vi "Helmholtz2D_FEM_Assemble.vi"(11 "Helmholtz2D FEM Data In":T1) -> (3 "Helmholtz2D FEM Data Out":T1)   [LabVIEW 2020, in "NI_PDE.lvlib"]
uses:
  <vilib>/gmath/NI_PDE.lvlib
  <vilib>/gmath/pde.llb/Helmholtz2D_FEM/Helmholtz2D_FEM_Data.ctl
  <vilib>/gmath/pde.llb/Common/PDE_Sparse Mtrx.ctl
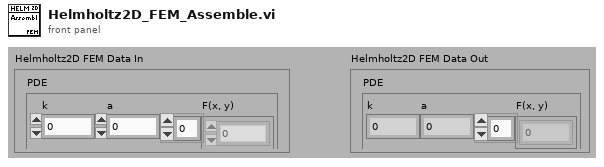
[diagram p1: front panel]
types:
  T1 = typedef "NI_PDE.lvlib/Helmholtz2D_FEM_Data.ctl" = cluster{"PDE":cluster{"k":dbl, "a":dbl, "F(x, y)":dbl[]}, "# of unknown":i32, "# of known":i32, "U(x, y)":dbl[], "X Used":dbl[], "Y Used":dbl[], "Triangulation":i32[][], "Coef Mtrx":T2}
  T2 = typedef "NI_PDE.lvlib/PDE_Sparse Mtrx.ctl" = cluster{"Row":cluster{"col":i32, "value":dbl}[]}[]
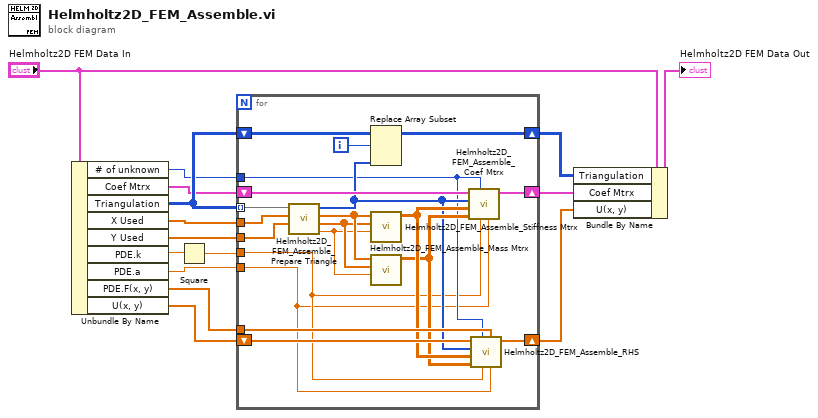
[diagram p0: block diagram]
diagram:
  n1 = Unbundle By Name("Helmholtz2D FEM Data In") -> ("# of unknown"=w11:i32, "Coef Mtrx"=w12:T2, "Triangulation"=w14:i32[][], "X Used"=w15:dbl[], "Y Used"=w13:dbl[], "PDE.k"=w8:dbl, "PDE.a"=w1:dbl, "PDE.F(x, y)"=w10:dbl[], "U(x, y)"=w9:dbl[])
  n2 = Square(x=w8) -> (x^2=w7:dbl)
  n3 = for {
    tunnel: w14 -> [w35] mode=indexing
    tunnel: w15 -> [w34]
    shift-right: [w31] -> w4
    shift-left: w14 -> [w32]
    tunnel: w13 -> [w33]
    shift-right: [w25] -> w3
    shift-left: w12 -> [w26]
    tunnel: w11 -> [w19]
    shift-right: [w16] -> w2
    shift-left: w9 -> [w24]
    tunnel: w10 -> [w23]
    tunnel: w7 -> [w18]
    tunnel: w1 -> [w17]
    i -> [w30]
    n4 = call <vilib>:"Helmholtz2D_FEM_Assemble_Prepare Triangle.vi"("Y"=w33, "X"=w34, "Triangle In"=w35) -> ("area"=w27:dbl, "Tri Y"=w28:dbl[], "Tri X"=w29:dbl[], "Triangle Out"=w20:i32[])  [unwired: 5 out]
    n5 = Replace Array Subset(array=w32, new element=w20, index (row)=w30) -> (w31:i32[][])  [unwired: 1 in]
    n6 = call <vilib>:"Helmholtz2D_FEM_Assemble_Stiffness Mtrx.vi"("area"=w27, "Tri Y"=w28, "Tri X"=w29) -> ("Stiffness Mtrx"=w22:dbl[][])  [unwired: 8 out]
    n7 = call <vilib>:"Helmholtz2D_FEM_Assemble_Mass Mtrx.vi"("area"=w27, "Tri Y"=w28, "Tri X"=w29) -> ("Mass Mtrx"=w21:dbl[][])  [unwired: 8 out]
    n8 = call <vilib>:"Helmholtz2D_FEM_Assemble_Coef Mtrx.vi"("a"=w17, "k"=w18, "# of unknown"=w19, "Mass Mtrx"=w21, "Stiffness Mtrx"=w22, "Triangle"=w20, "Coef Mtrx In"=w26) -> ("Coef Mtrx Out"=w25:T2)  [unwired: 4 out]
    n9 = call <vilib>:"Helmholtz2D_FEM_Assemble_RHS.vi"("a"=w17, "F(x, y)"=w23, "k"=w18, "# of unknown"=w19, "Mass Mtrx"=w21, "Stiffness Mtrx"=w22, "Triangle"=w20, "RHS In"=w24) -> ("RHS Out"=w16:dbl[])  [unwired: 3 out]
  }
  n10 = Bundle By Name(cluster="Helmholtz2D FEM Data In", "Triangulation"=w4, "Coef Mtrx"=w3, "U(x, y)"=w2) -> (→"Helmholtz2D FEM Data Out":T1)
